vi "PID Timing Estimation.vi"(7 "R":bool, 10 "dt (s) in":dbl=-1.0, 11 "PID Timing Estimation in":refnum<class "PID Timing Estimation.lvclass">) -> (2 "dt (s) out":dbl, 3 "PID Timing Estimation out":refnum<class "PID Timing Estimation.lvclass">)   [LabVIEW 2019, in "control.lvlib" / "PID Timing Estimation.lvclass"]
uses:
  PID Timing Estimation.lvclass
  PID Timing Estimation.lvclass/PID Timing Estimation.ctl
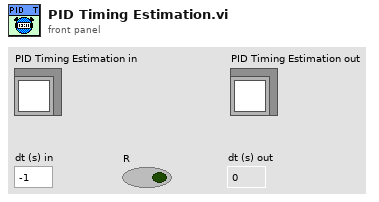
[diagram p1: front panel]
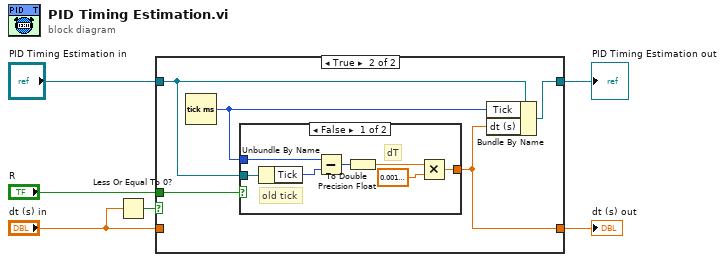
[diagram p0: block diagram]
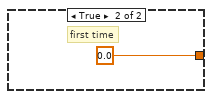
[diagram p3: hidden frame]
diagram:
  n1 = Less Or Equal To 0?(x="dt (s) in") -> (x <= 0?=w1:bool)
  n2 = case shown="True" w1 {
    tunnel: "dt (s) in" -> [w8 _]
    tunnel: "R" -> [_ w13]
    tunnel: [w8 w12] -> w2
    tunnel: "PID Timing Estimation in" -> [w7 w10]
    tunnel: [w7 w9] -> w5
    frame False {
      # "Ext dt"
    }
    frame True {
      n3 = Tick Count (ms)() -> (millisecond timer value=w11:u32)
      n4 = case shown="False" w13 {
        tunnel: [w16 0.0] -> w12
        tunnel: w11 -> [w20 _]
        tunnel: w10 -> [w15 _]
        frame False {
          # "old tick"
          # "dT"
          n5 = Unbundle By Name(w15) -> ("Tick"=w14:u32)
          n6 = Subtract(x=w20, y=w14) -> (x-y=w17:u32)
          n7 = To Double Precision Float(number=w17) -> (double precision float=w18:dbl)
          n8 = Multiply(x=w18, y=0.0010000000474974513) -> (x*y=w16:dbl)
        }
        frame True {
          # "first time"
        }
      }
      n9 = Bundle By Name(cluster=w10, "Tick"=w11, "dt (s)"=w12) -> (w9:refnum<class "PID Timing Estimation.lvclass">)
    }
  }
  "PID Timing Estimation out" <- w5
  "dt (s) out" <- w2
